vi "Quit.vi"(8 "error in (no error)":errorcluster, 11 "Tree in":refnum<class "Tree.lvclass">) -> (0 "error out":errorcluster, 3 "Tree out":refnum<class "Tree.lvclass">)   [LabVIEW 2012, in "MDSplus.lvlib" / "Tree.lvclass"]
doc: "Quit editing session."
uses:
  <vilib>/MDSplus/Classes/Tree_Class/Tree.lvclass
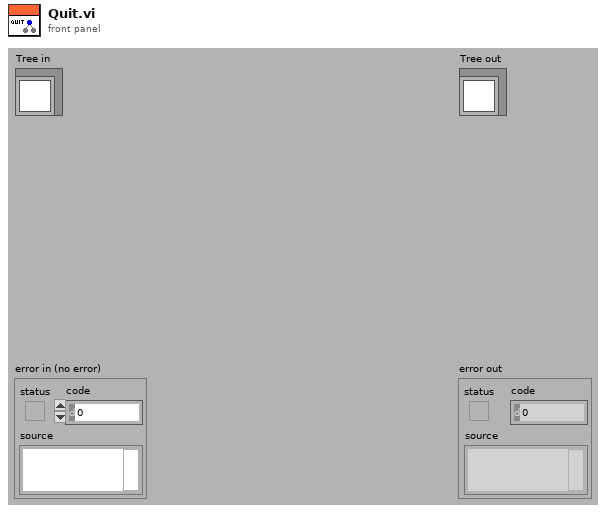
[diagram p1: front panel]
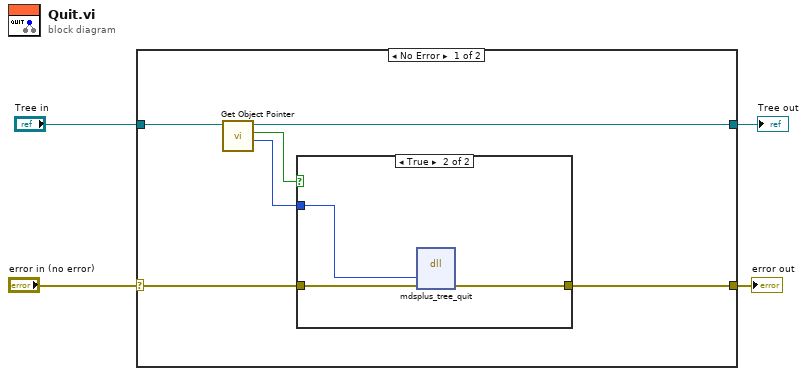
[diagram p0: block diagram]
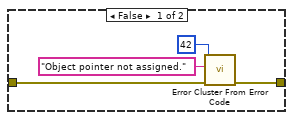
[diagram p2: hidden frame]
diagram:
  n1 = case shown="No Error" "error in (no error)" {
    selector: "error in (no error)" -> [w7 w19]
    tunnel: [w8 w19] -> w3
    tunnel: [w9 w18] -> w1
    tunnel: "Tree in" -> [w10 w18]
    frame No Error {
      n2 = call-dynamic "Get Object Pointer.vi"("Tree in"=w10) -> ("Object Pointer"=w5:i64, "Assigned object pointer?"=w6:bool, "Tree out"=w9:refnum<class "Tree.lvclass">)  [unwired: 8 in]
      n3 = case shown="True" w6 {
        tunnel: [w11 w17] -> w8
        tunnel: w7 -> [w12 w16]
        tunnel: w5 -> [_ w15]
        frame False {
          n4 = call <vilib>:"Error Cluster From Error Code.vi"("error in (no error)"=w12, "error message (\"\")"="Object pointer not assigned." ("error message (\"\")"), "error code (0)"=42) -> ("error out"=w11:errorcluster)  [unwired: 6 in]
        }
        frame True {
          n5 = dll-call lib="MDSobjectsLVShr" fn="mdsplus_tree_quit"("lvTreePtr"=w15, "error"=w16) -> ("error"=w17:errorcluster)  [unwired: 5 in, 2 out]
        }
      }
    }
    frame Error {
    }
  }
  "error out" <- w3
  "Tree out" <- w1
